vi "Parse Single Channel.vi"(10 "Raw Data":u8[](array[numeric])) -> (2 "Channel":T1)   [LabVIEW 2018, in "Control Box.lvlib" / "Control Box.lvclass"]
uses:
  Control Box.lvclass
  Custom Controls/Channel Status.ctl
  Control Box.lvlib
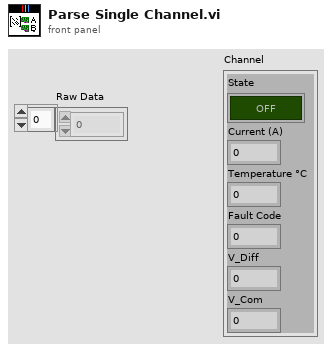
[diagram p1: front panel]
types:
  T1 = typedef "Control Box.lvlib/Channel Status.ctl" = cluster{"State":bool, "Current (A)":dbl, "Temperature °C":dbl, "Fault Code":u8, "V_Diff":dbl, "V_Com":dbl}
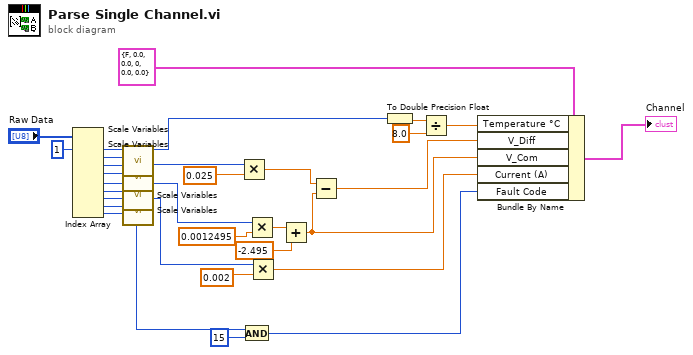
[diagram p0: block diagram]
diagram:
  n1 = Index Array(array="Raw Data", index #1=1 ("index")) -> (element #1=w27:u8, element #2=w26:u8, element #3=w25:u8, element #4=w24:u8, element #5=w23:u8, element #6=w22:u8, element #7=w21:u8, element #8=w20:u8, element #9=w9:u8)  [unwired: 8 in]
  n2 = call "Scale Variables.vi"("Var 2"=w26, "Var 1"=w27) -> ("Scaled output"=w19:i16)  [unwired: 9 in]
  n3 = call "Scale Variables.vi"("Var 2"=w24, "Var 1"=w25) -> ("Scaled output"=w15:i16)  [unwired: 9 in]
  n4 = call "Scale Variables.vi"("Var 2"=w22, "Var 1"=w23) -> ("Scaled output"=w13:i16)  [unwired: 9 in]
  n5 = call "Scale Variables.vi"("Var 2"=w20, "Var 1"=w21) -> ("Scaled output"=w12:i16)  [unwired: 9 in]
  n6 = Multiply(x=w15, y=0.025) -> (x*y=w7:dbl)
  n7 = And(x=w9, y=u8 15) -> (x .and. y?=w2:u8)
  n8 = Multiply(x=w13, y=0.0012495) -> (x*y=w6:dbl)
  n9 = Multiply(x=w12, y=0.002) -> (x*y=w3:dbl)
  n10 = Add(x=w6, y=-2.495) -> (x+y=w4:dbl)
  n11 = Subtract(x=w7, y=w4) -> (x-y=w5:dbl)
  n12 = To Double Precision Float(number=w19) -> (double precision float=w18:dbl)
  n13 = Divide(x=w18, y=8.0) -> (x/y=w16:dbl)
  n14 = Bundle By Name(cluster=T1 {"State"=FALSE, "Current (A)"=0.0, "Temperature °C"=0.0, "Fault Code"=0, "V_Diff"=0.0, "V_Com"=0.0} ("Channel"), "Temperature °C"=w16, "V_Diff"=w5, "V_Com"=w4, "Current (A)"=w3, "Fault Code"=w2) -> (→"Channel":T1)
